vi "Airmar Interpret NMEA Sentence.vi"(11 "NMEA Sentence":string) -> ()   [LabVIEW 2013]
doc: "Interprets the NMEA 0813 sentences that we are using from our Airmar PB200 WeatherStation sensor.\nBy Jaime McCandless\nTODO: finish implementing NMEA sentences"
uses:
  <vilib>/regexp/Match Regular Expression.xnode
  trunk/Software/2-Think/2 Globals/2 Global.vi
  Data/TypeDefs/UTM Location.ctl
  Data/TypeDefs/GPS Sensor Status.ctl
panel:
  out "Estimated error":dbl
  in  "UTC Time Zone":i32=-5
  in  "Tab Control":T1(tab)
  out "GPS (GGA) Data":T2
  out "GPS (GLL) Data":T3
  out "GPGSA Data":T4
  out "UTC Time":timestamp
  out "Local Time":timestamp
  out "Lattitude (ddmm.mmmm)":dbl format="%_8g"
  out "Lattitude North/South":string
  out "Longitude (ddmm.mmmm)":dbl format="%_8g"
  out "Longitude East/West":string
  out "Speed over ground (knots)":dbl format="%_3g"
  out "Course over ground (degrees)":dbl format="%_4g"
  out "Magnetic Variation (degrees)":dbl format="%_4g"
  out "Variation East/West":string
  out "GPS (RMC) Data":T5 {"Course over ground (degrees)" format="%#.6g"; "Speed over ground (knots)" format="%#.6g"; "Magnetic Variation (degrees)" format="%#.6g"; "Longitude (ddmm.mmmm)" format="%#.6g"; "Lattitude (ddmm.mmmm)" format="%#.6g"}
  out "GPS Data Valid?":bool
  out "Robot UTM Location":T6 {"North" format="%#_10f"; "East" format="%#_8f"}
  out "GPS (VTG) Data":T7
  out "Heading":dbl
  out "Turn (ROT) Data":T8
  out "Meteorological Data":T9
  out "Theoretical true wind direction":T10(graph)
  out "Relative wind direction":cluster{dbl, "Filtered Value Out":dbl}(graph)
  out "Wind (MWV) Data, Theoretical":T11
  out "Wind (MWV) Data, Relative":T11
  out "Transducer (XDR) B Data":cluster{"Pitch (deg)":dbl, "Roll (deg)":dbl}
  out "Transducer (XDR) A Data":T12
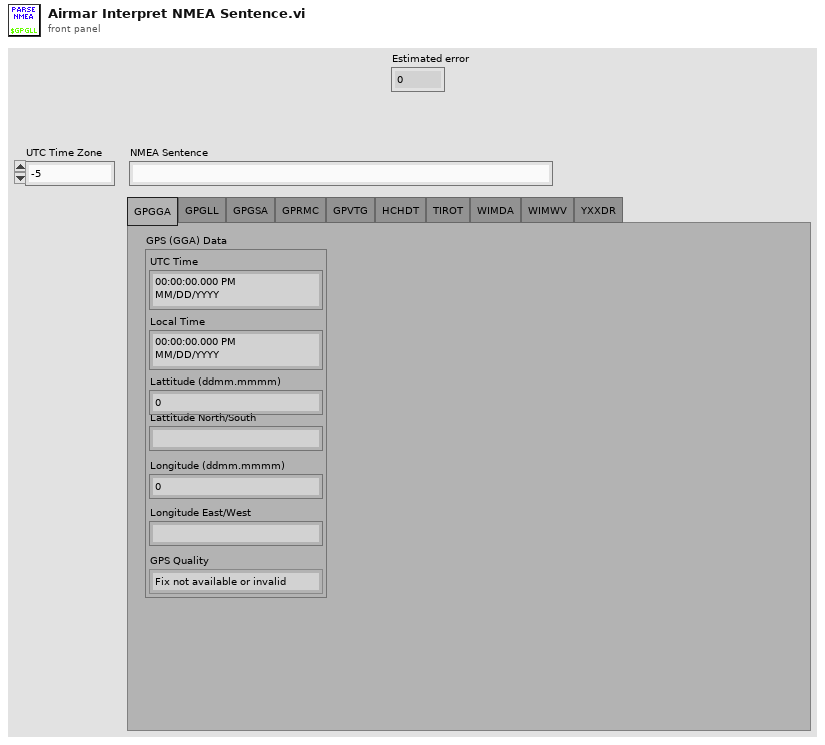
[diagram p1: front panel]
types:
  T1 = enum32{"GPGGA", "GPGLL", "GPGSA", "GPRMC", "GPVTG", "HCHDT", "TIROT", "WIMDA", "WIMWV", "YXXDR"}
  T2 = cluster{"UTC Time":timestamp, "Local Time":timestamp, "Lattitude (ddmm.mmmm)":dbl, "Lattitude North/South":string, "Longitude (ddmm.mmmm)":dbl, "Longitude East/West":string, "GPS Quality":enum16{"Fix not available or invalid", "GPS SPS Mode, fix valid", "Differential GPS, SPS Mode, fix valid", "GPS PPS Mode, fix valid", "Real Time Kinematic (RTK)", "Float RTK", "Estimated (dead reckoning) Mode", "Manual Input Mode", "Simulator Mode"}}
  T3 = cluster{"UTC Time":timestamp, "Local Time":timestamp, "Lattitude (ddmm.mmmm)":dbl, "Lattitude North/South":string, "Longitude (ddmm.mmmm)":dbl, "Longitude East/West":string, "GPS Mode":string, "GPS Data Valid?":bool}
  T4 = cluster{"Mode":string, "Fix Strength":i32, "Satellite IDs":i32[], "PDOP":dbl, "HDOP":dbl, "VDOP":dbl}
  T5 = cluster{"UTC Time":timestamp, "Local Time":timestamp, "Lattitude (ddmm.mmmm)":dbl, "Lattitude North/South":string, "Longitude (ddmm.mmmm)":dbl, "Longitude East/West":string, "Magnetic Variation (degrees)":dbl, "Variation East/West":string, "Speed over ground (knots)":dbl, "Course over ground (degrees)":dbl}
  T6 = typedef "UTM Location.ctl" = cluster{"UTM Zone":dbl, "Hemisphere":enum16{"North", "South"}, "East":dbl, "North":dbl}
  T7 = cluster{"Course Over Ground (True)":dbl, "Course Over Ground (Magnetic)":dbl, "Speed Over Ground (Knots)":dbl, "Speed Over Ground (km/hr)":dbl, "GPS Mode":string}
  T8 = cluster{"Rate of Turn (deg/min)":dbl, "Turn Rotation Data Valid?":bool}
  T9 = cluster{"Barometric Pressure (inches of mercury)":dbl, "Barometric Pressure (bars)":dbl, "Air temperature (degC)":dbl, "Relative humidity (%)":dbl, "Wind direction, True (deg)":dbl, "Wind direction, Magnetic (deg)":dbl, "Wind speed (knots)":dbl, "Wind speed (m/s)":dbl}
  T10 = cluster{"Robot\nHeading ":dbl, "Robot\nHeading ":dbl}
  T11 = cluster{"Angle relative to boat (deg)":dbl, "Wind Data Valid?":bool, "Wind speed (knots)":dbl, "True (T) or Relative (R)":string}
  T12 = cluster{"Calc. Relative Wind Chill (degC)":dbl, "Calc. Theoretical Wind Chill (degC)":dbl, "Calc. Heat Index (degC)":dbl, "Meas. Barometric Pressure (bars)":dbl}
  T13 = cluster{"second":i32, "minute":i32, "hour":i32, "day of month":i32, "month":i32, "year":i32, "day of week":i32, "day of year":i32, "is DST":i32}
  T14 = typedef "GPS Sensor Status.ctl" = cluster{"Sensor Connected":bool, "Sensor OK":bool, "GPS Lock":bool, "Sensor Initialized":bool}
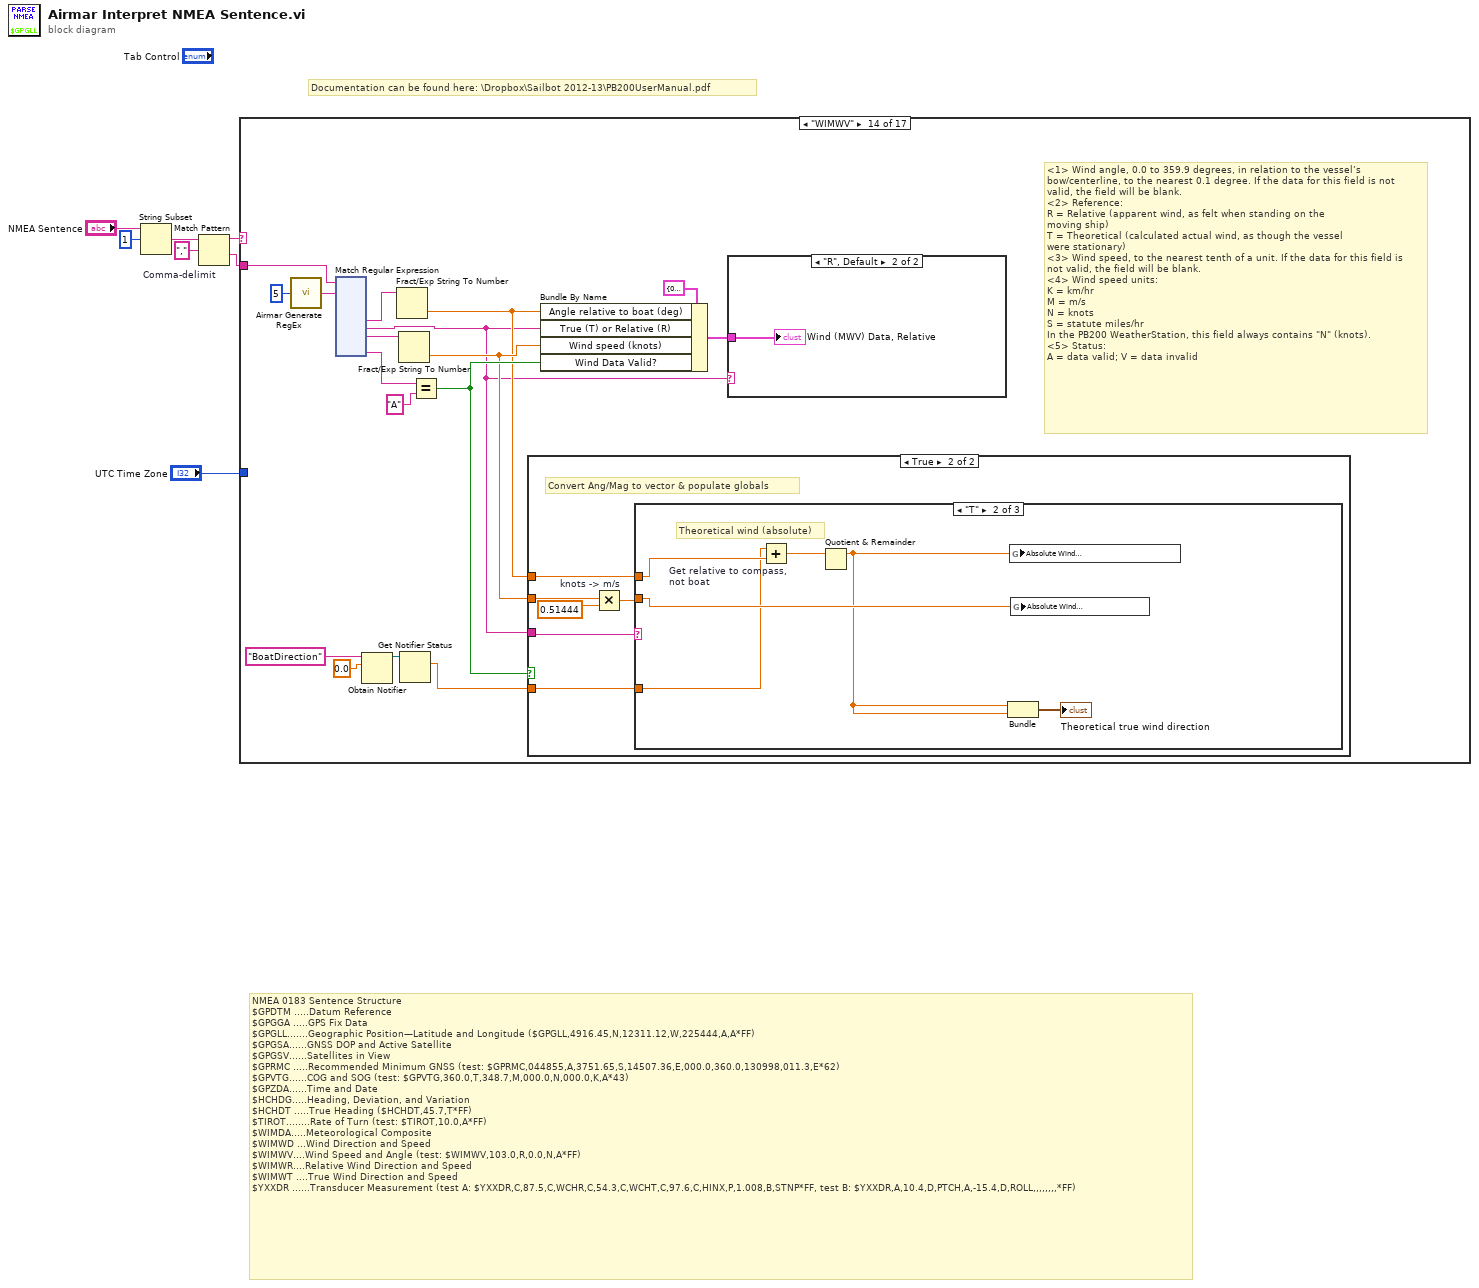
[diagram p0: block diagram]
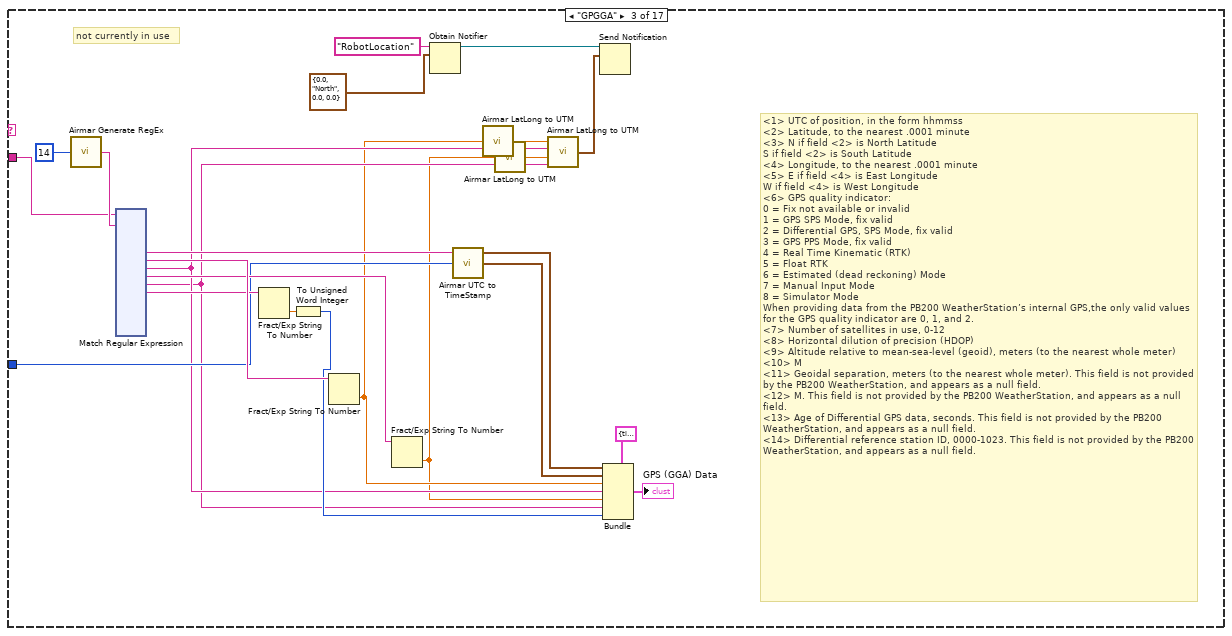
[diagram p4: hidden frame]
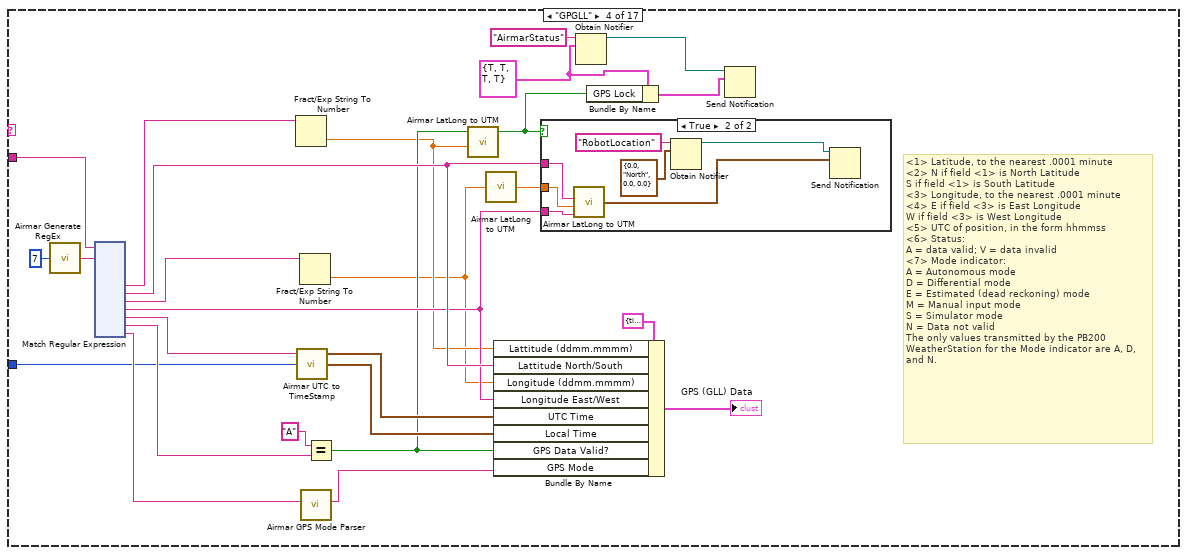
[diagram p5: hidden frame]
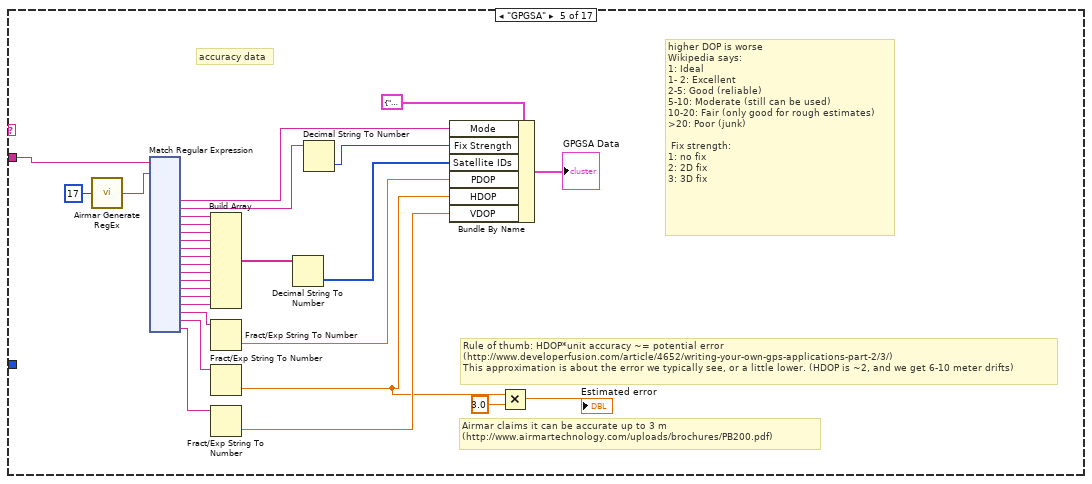
[diagram p7: hidden frame]
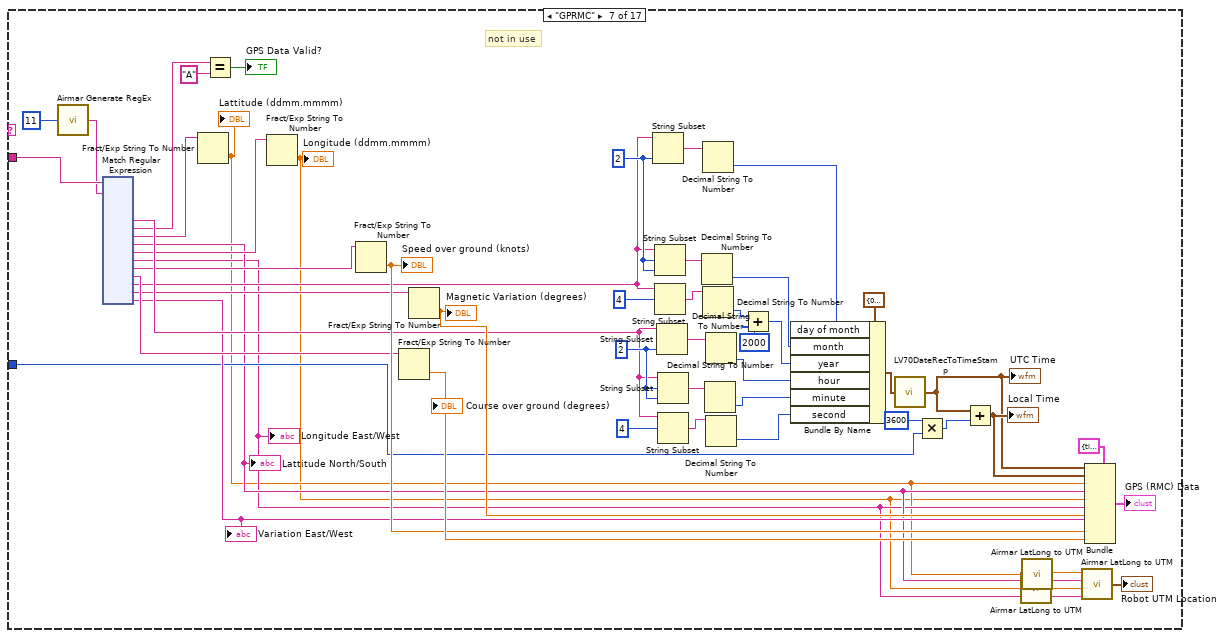
[diagram p9: hidden frame]
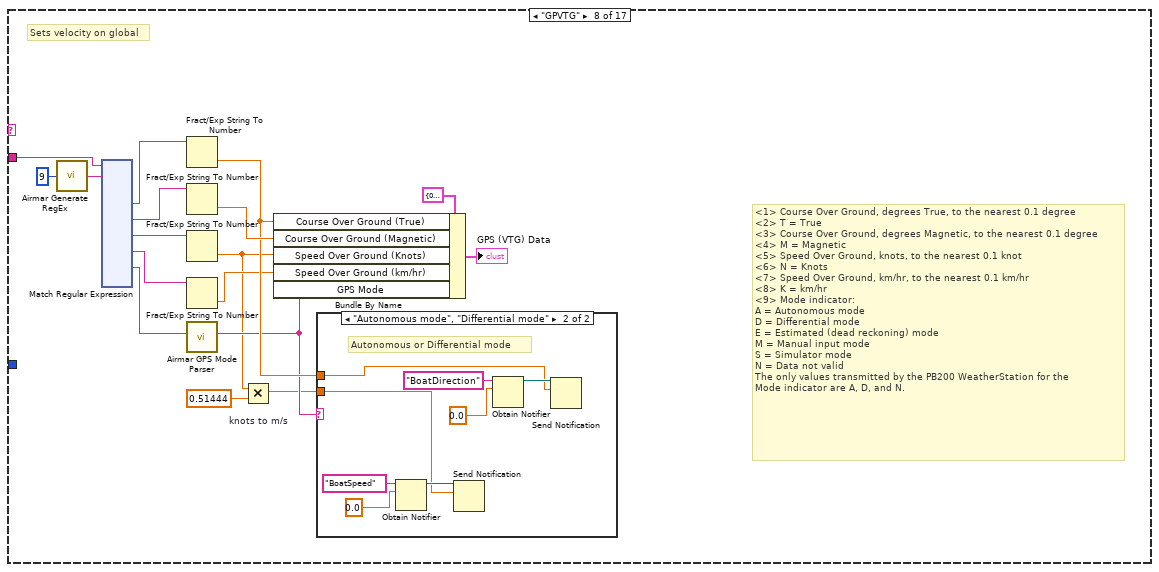
[diagram p10: hidden frame]
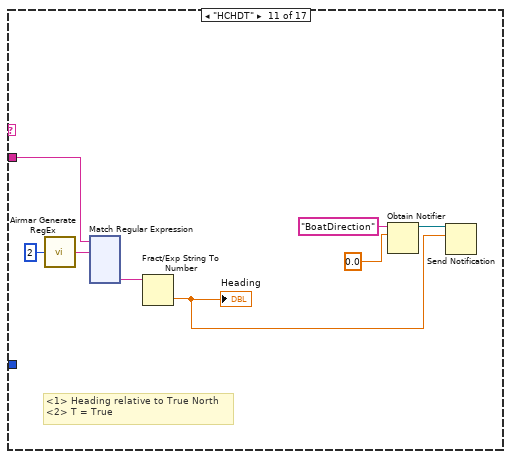
[diagram p14: hidden frame]
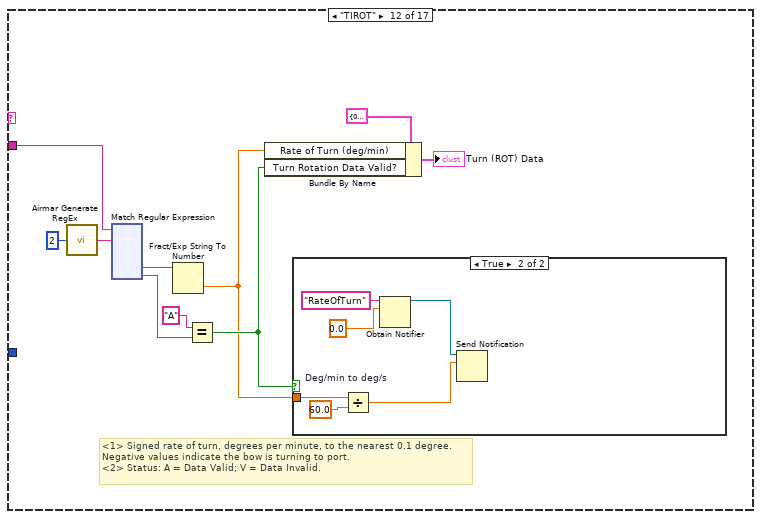
[diagram p15: hidden frame]
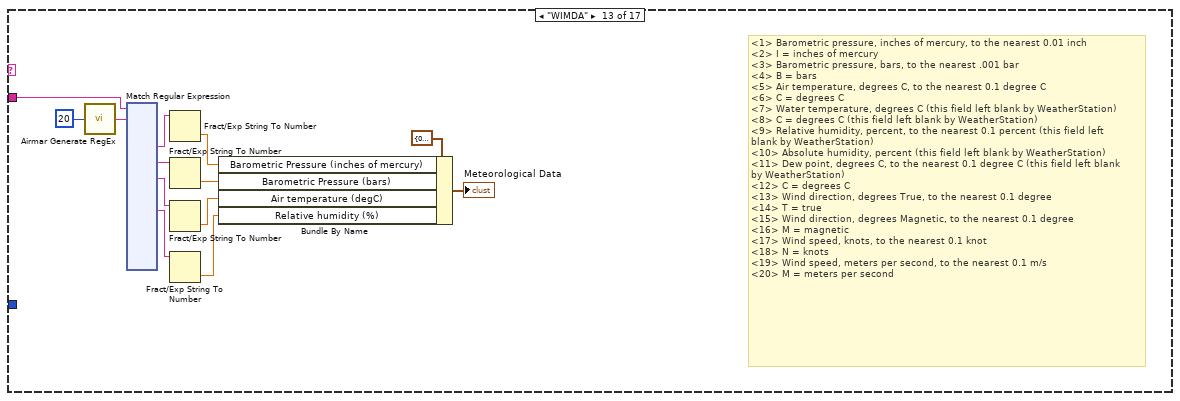
[diagram p17: hidden frame]
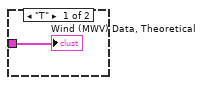
[diagram p18: hidden frame]
diagram:
  # "Documentation can be found here: \\Dropbox\\Sailbot 2012-13\\PB200UserManual.pdf"
  # "NMEA 0183 Sentence Structure\n$GPDTM .....Datum Reference\n$GPGGA .....GPS Fix Data\n$GPGLL.......Geographic Position—Latitude and Longitude ($GPGLL,4916.45,N,12311.12,W,225444,A,A*FF)\n$GPGSA......GNSS DOP and Active Satellite\n$GPGSV......Satellites in View\n$GPRMC .....Recommended Minimum GNSS (test: $GPRMC,044855,A,3751.65,S,14507.36,E,000.0,360.0,130998,011.3,E*62)\n$GPVTG......COG and SOG (test: $GPVTG,360.0,T,348.7,M,000.0,N,000.0,K,A*43)\n$GPZDA......Time and Date\n$HCHDG.....Heading, Deviation, and Variation\n$HCHDT .....True Heading ($HCHDT,45.7,T*FF)\n$TIROT........Rate of Turn (test: $TIROT,10.0,A*FF)\n$WIMDA.....Meteorological Composite\n$WIMWD ...Wind Direction and Speed\n$WIMWV....Wind Speed and Angle (test: $WIMWV,103.0,R,0.0,N,A*FF)\n$WIMWR....Relative Wind Direction and Speed\n$WIMWT ....True Wind Direction and Speed\n$YXXDR ......Transducer Measurement (test A: $YXXDR,C,87.5,C,WCHR,C,54.3,C,WCHT,C,97.6,C,HINX,P,1.008,B,STNP*FF, test B: $YXXDR,A,10.4,D,PTCH,A,-15.4,D,ROLL,,,,,,,,*FF)"
  n1 = String Subset(string="NMEA Sentence", offset (0)=1) -> (substring=w4:string)  [unwired: 1 in]
  n2 = Match Pattern "Comma-delimit"(string=w4, regular expression=",") -> (before substring=w5:string, after substring=w6:string)  [unwired: 1 in, 2 out]
  n3 = case shown="\"WIMWV\"" w5 {
    tunnel: w6 -> [_ _ w29 w174 w335 _ w484 w653 _ _ w792 w914 w1048 w1191 _ _ w1330]
    tunnel: "UTC Time Zone" -> [_ _ w18 w166 _ _ w472 _ _ _ _ _ _ _ _ _ _]
    frame "", Default {
    }
    frame "GPDTM" {
      # "unimplemented"
    }
    frame "GPGGA" {
      # "not currently in use"
      # "<1> UTC of position, in the form hhmmss\n<2> Latitude, to the nearest .0001 minute\n<3> N if field <2> is North Latitude\nS if field <2> is South Latitude\n<4> Longitude, to the nearest .0001 minute\n<5> E if field <4> is East Longitude\nW if field <4> is West Longitude\n<6> GPS quality indicator:\n0 = Fix not available or invalid\n1 = GPS SPS Mode, fix valid\n2 = Differential GPS, SPS Mode, fix valid\n3 = GPS PPS Mode, fix valid\n4 = Real Time Kinematic (RTK)\n5 = Float RTK\n6 = Estimated (dead reckoning) Mode\n7 = Manual Input Mode\n8 = Simulator Mode\nWhen providing data from the PB200 WeatherStation’s internal GPS,the only valid values for the GPS quality indicator are 0, 1, and 2.\n<7> Number of satellites in use, 0-12\n<8> Horizontal dilution of precision (HDOP)\n<9> Altitude relative to mean-sea-level (geoid), meters (to the nearest whole meter)\n<10> M\n<11> Geoidal separation, meters (to the nearest whole meter). This field is not provided by the PB200 WeatherStation, and appears as a null field.\n<12> M. This field is not provided by the PB200 WeatherStation, and appears as a null field.\n<13> Age of Differential GPS data, seconds. This field is not provided by the PB200 WeatherStation, and appears as a null field.\n<14> Differential reference station ID, 0000-1023. This field is not provided by the PB200 WeatherStation, and appears as a null field."
      n4 = call "Airmar Generate RegEx.vi"("# Datums"=14) -> ("RegEx"=w30:string)
      n5 = xnode "Match Regular Expression"("input string"=w29, "regular expression"=w30) -> ("submatch 1"=w21:string, "submatch 2"=w27:string, "submatch 3"=w17:string, "submatch 4"=w26:string, "submatch 5"=w16:string, "submatch 6"=w25:string)  [unwired: 4 in, 10 out]
      n6 = Fract/Exp String To Number(string=w25) -> (number=w24:dbl)  [unwired: 3 in, 1 out]
      n7 = To Unsigned Word Integer(number=w24) -> (unsigned 16bit integer=w23:u16)
      n8 = Fract/Exp String To Number(string=w27) -> (number=w14:dbl)  [unwired: 3 in, 1 out]
      n9 = Fract/Exp String To Number(string=w26) -> (number=w12:dbl)  [unwired: 3 in, 1 out]
      n10 = Obtain Notifier(name (unnamed)="RobotLocation", notification data type=T6 {"UTM Zone"=0.0, "Hemisphere"=enum."North", "East"=0.0, "North"=0.0} ("UTM Location")) -> (notifier out=w9:refnum<notifier>)  [unwired: 2 in, 2 out]
      n11 = call "Airmar UTC to TimeStamp.vi"("UTC Time Zone in"=w18, "UTC (hhmmss)"=w21) -> ("Local Time"=w19:timestamp, "UTC Time"=w20:timestamp)  [unwired: 2 in]
      n12 = call "Airmar LatLong to UTM.vi"("Lattitude/Longitude in ddmm.mmmm"=w14) -> ("Latitude/Longitude in dd.dddddd"=w15:dbl)
      n13 = call "Airmar LatLong to UTM.vi"("Lattitude/Longitude in ddmm.mmmm"=w12) -> ("Latitude/Longitude in dd.dddddd"=w13:dbl)
      n14 = call "Airmar LatLong to UTM.vi"("East/West"=w16, "Longitude"=w13, "North/South"=w17, "Latitude"=w15) -> ("Robot UTM Location"=w8:T6)
      n15 = Send Notification(notification=w8, notifier=w9) -> ()  [unwired: 1 in, 2 out]
      n16 = Bundle(cluster=T2 {"UTC Time"=timestamp(0 s since 1904-01-01), "Local Time"=timestamp(0 s since 1904-01-01), "Lattitude (ddmm.mmmm)"=0.0, "Lattitude North/South"="", "Longitude (ddmm.mmmm)"=0.0, "Longitude East/West"="", "GPS Quality"=enum."GPS SPS Mode, fix valid"} ("Cluster"), "UTC Time"=w20, "Local Time"=w19, "Lattitude (ddmm.mmmm)"=w14, "Lattitude North/South"=w17, "Longitude (ddmm.mmmm)"=w12, "Longitude East/West"=w16, "GPS Quality"=w23) -> (→"GPS (GGA) Data":T2)
    }
    frame "GPGLL" {
      w157 = T14 {"Sensor Connected"=TRUE, "Sensor OK"=TRUE, "GPS Lock"=TRUE, "Sensor Initialized"=TRUE} ("input cluster")
      # "<1> Latitude, to the nearest .0001 minute\n<2> N if field <1> is North Latitude\nS if field <1> is South Latitude\n<3> Longitude, to the nearest .0001 minute\n<4> E if field <3> is East Longitude\nW if field <3> is West Longitude\n<5> UTC of position, in the form hhmmss\n<6> Status:\nA = data valid; V = data invalid\n<7> Mode indicator:\nA = Autonomous mode\nD = Differential mode\nE = Estimated (dead reckoning) mode\nM = Manual input mode\nS = Simulator mode\nN = Data not valid\nThe only values transmitted by the PB200 WeatherStation for the Mode indicator are A, D, and N."
      n17 = call "Airmar Generate RegEx.vi"("# Datums"=7) -> ("RegEx"=w178:string)
      n18 = xnode "Match Regular Expression"("input string"=w174, "regular expression"=w178) -> ("submatch 1"=w177:string, "submatch 2"=w164:string, "submatch 3"=w176:string, "submatch 4"=w163:string, "submatch 5"=w173:string, "submatch 6"=w169:string, "submatch 7"=w175:string)  [unwired: 4 in, 5 out]
      n19 = Fract/Exp String To Number(string=w177) -> (number=w161:dbl)  [unwired: 3 in, 1 out]
      n20 = call "Airmar UTC to TimeStamp.vi"("UTC Time Zone in"=w166, "UTC (hhmmss)"=w173) -> ("Local Time"=w168:timestamp, "UTC Time"=w167:timestamp)  [unwired: 2 in]
      n21 = Fract/Exp String To Number(string=w176) -> (number=w160:dbl)  [unwired: 3 in, 1 out]
      n22 = call "Airmar GPS Mode Parser.vi"("GPS Mode (Char)"=w175) -> ("GPS Mode (Description)"=w171:string)  [unwired: 6 in]
      n23 = Equal?(x="A" ("y"), y=w169) -> (x = y?=w162:bool)
      n24 = call "Airmar LatLong to UTM.vi"("Longitude"=w161) -> ()  [unwired: 3 in, 1 out]
      n25 = call "Airmar LatLong to UTM.vi"("Lattitude/Longitude in ddmm.mmmm"=w160) -> ("Latitude/Longitude in dd.dddddd"=w159:dbl)
      n26 = Bundle By Name(cluster=T3 {"UTC Time"=timestamp(0 s since 1904-01-01), "Local Time"=timestamp(0 s since 1904-01-01), "Lattitude (ddmm.mmmm)"=0.0, "Lattitude North/South"="", "Longitude (ddmm.mmmm)"=0.0, "Longitude East/West"="", "GPS Mode"="", "GPS Data Valid?"=FALSE} ("Cluster"), "Lattitude (ddmm.mmmm)"=w161, "Lattitude North/South"=w164, "Longitude (ddmm.mmmm)"=w160, "Longitude East/West"=w163, "UTC Time"=w167, "Local Time"=w168, "GPS Data Valid?"=w162, "GPS Mode"=w171) -> (→"GPS (GLL) Data":T3)
      n27 = case shown="True" w162 {
        tunnel: w164 -> [_ w186]
        tunnel: w159 -> [_ w185]
        tunnel: w163 -> [_ w184]
        frame False {
        }
        frame True {
          n28 = call "Airmar LatLong to UTM.vi"("East/West"=w184, "Longitude"=w185, "North/South"=w186) -> ("Robot UTM Location"=w183:T6)  [unwired: 1 in]
          n29 = Obtain Notifier(name (unnamed)="RobotLocation", notification data type=T6 {"UTM Zone"=0.0, "Hemisphere"=enum."North", "East"=0.0, "North"=0.0} ("UTM Location")) -> (notifier out=w180:refnum<notifier>)  [unwired: 2 in, 2 out]
          n30 = Send Notification(notification=w183, notifier=w180) -> ()  [unwired: 1 in, 2 out]
        }
      }
      n31 = Obtain Notifier(name (unnamed)="AirmarStatus", notification data type=w157) -> (notifier out=w156:refnum<notifier>)  [unwired: 2 in, 2 out]
      n32 = Bundle By Name(cluster=w157, "GPS Lock"=w162) -> (w155:T14)
      n33 = Send Notification(notification=w155, notifier=w156) -> ()  [unwired: 1 in, 2 out]
    }
    frame "GPGSA" {
      # "Airmar claims it can be accurate up to 3 m\n(http://www.airmartechnology.com/uploads/brochures/PB200.pdf)"
      # "Rule of thumb: HDOP*unit accuracy ~= potential error\n(http://www.developerfusion.com/article/4652/writing-your-own-gps-applications-part-2/3/)\nThis approximation is about the error we typically see, or a little lower. (HDOP is ~2, and we get 6-10 meter drifts)"
      # "higher DOP is worse\nWikipedia says:\n1: Ideal\n1- 2: Excellent\n2-5: Good (reliable)\n5-10: Moderate (still can be used)\n10-20: Fair (only good for rough estimates)\n>20: Poor (junk)\n\n Fix strength: \n1: no fix\n2: 2D fix\n3: 3D fix"
      # "accuracy data"
      n34 = call "Airmar Generate RegEx.vi"("# Datums"=17) -> ("RegEx"=w334:string)
      n35 = xnode "Match Regular Expression"("input string"=w335, "regular expression"=w334) -> ("submatch 1"=w331:string, "submatch 2"=w330:string, "submatch 3"=w328:string, "submatch 4"=w327:string, "submatch 5"=w326:string, "submatch 6"=w325:string, "submatch 7"=w324:string, "submatch 8"=w323:string, "submatch 9"=w322:string, "submatch 10"=w321:string, "submatch 11"=w320:string, "submatch 12"=w319:string, "submatch 13"=w318:string, "submatch 14"=w317:string, "submatch 15"=w314:string, "submatch 16"=w312:string, "submatch 17"=w311:string)  [unwired: 4 in, 5 out]
      n36 = Build Array(w328, w327, w326, w325, w324, w323, w322, w321, w320, w319, w318, w317) -> (w316:string[])
      n37 = Fract/Exp String To Number(string=w314) -> (number=w313:dbl)  [unwired: 3 in, 1 out]
      n38 = Fract/Exp String To Number(string=w312) -> (number=w308:dbl)  [unwired: 3 in, 1 out]
      n39 = Fract/Exp String To Number(string=w311) -> (number=w310:dbl)  [unwired: 3 in, 1 out]
      n40 = Decimal String To Number(string=w316) -> (number=w315:i32[])  [unwired: 2 in, 1 out]
      n41 = Decimal String To Number(string=w330) -> (number=w329:i32)  [unwired: 2 in, 1 out]
      n42 = Bundle By Name(cluster=T4 {"Mode"="", "Fix Strength"=0, "Satellite IDs"=[], "PDOP"=0.0, "HDOP"=0.0, "VDOP"=0.0} ("GPGSA Data"), "Mode"=w331, "Fix Strength"=w329, "Satellite IDs"=w315, "PDOP"=w313, "HDOP"=w308, "VDOP"=w310) -> (→"GPGSA Data":T4)
      n43 = Multiply(x=w308, y=3.0) -> (x*y=→"Estimated error":dbl)
    }
    frame "GPGSV" {
      # "unimplemented"
    }
    frame "GPRMC" {
      w502 = 2 ("length (rest)")
      w492 = 2 ("length (rest)")
      # "not in use"
      n44 = call "Airmar Generate RegEx.vi"("# Datums"=11) -> ("RegEx"=w474:string)
      n45 = xnode "Match Regular Expression"("input string"=w484, "regular expression"=w474) -> ("submatch 1"=w483:string, "submatch 2"=w482:string, "submatch 3"=w481:string, "submatch 4"=w471:string, "submatch 5"=w480:string, "submatch 6"=w470:string, "submatch 7"=w479:string, "submatch 8"=w478:string, "submatch 9"=w477:string, "submatch 10"=w476:string, "submatch 11"=w475:string)  [unwired: 4 in, 5 out]
      "Lattitude North/South" <- w471
      "Longitude East/West" <- w470
      "Variation East/West" <- w475
      n46 = Fract/Exp String To Number(string=w481) -> (number=w467:dbl)  [unwired: 3 in, 1 out]
      "Lattitude (ddmm.mmmm)" <- w467
      n47 = Equal?(x=w482, y="A") -> (x = y?=→"GPS Data Valid?":bool)
      n48 = Fract/Exp String To Number(string=w480) -> (number=w465:dbl)  [unwired: 3 in, 1 out]
      "Longitude (ddmm.mmmm)" <- w465
      n49 = Fract/Exp String To Number(string=w479) -> (number=w512:dbl)  [unwired: 3 in, 1 out]
      "Speed over ground (knots)" <- w512
      n50 = Fract/Exp String To Number(string=w478) -> (number=w513:dbl)  [unwired: 3 in, 1 out]
      "Course over ground (degrees)" <- w513
      n51 = Fract/Exp String To Number(string=w476) -> (number=w511:dbl)  [unwired: 3 in, 1 out]
      "Magnetic Variation (degrees)" <- w511
      n52 = String Subset(string=w477, length (rest)=w502) -> (substring=w503:string)  [unwired: 1 in]
      n53 = String Subset(string=w477, offset (0)=w502, length (rest)=w502) -> (substring=w501:string)
      n54 = String Subset(string=w477, offset (0)=4) -> (substring=w499:string)  [unwired: 1 in]
      n55 = String Subset(string=w483, length (rest)=w492) -> (substring=w488:string)  [unwired: 1 in]
      n56 = String Subset(string=w483, offset (0)=w492, length (rest)=w492) -> (substring=w494:string)
      n57 = String Subset(string=w483, offset (0)=4) -> (substring=w496:string)  [unwired: 1 in]
      n58 = Decimal String To Number(string=w501) -> (number=w505:i32)  [unwired: 2 in, 1 out]
      n59 = Decimal String To Number(string=w503) -> (number=w504:i32)  [unwired: 2 in, 1 out]
      n60 = Decimal String To Number(string=w499) -> (number=w506:i32)  [unwired: 2 in, 1 out]
      n61 = Decimal String To Number(string=w494) -> (number=w493:i32)  [unwired: 2 in, 1 out]
      n62 = Decimal String To Number(string=w488) -> (number=w491:i32)  [unwired: 2 in, 1 out]
      n63 = Decimal String To Number(string=w496) -> (number=w497:i32)  [unwired: 2 in, 1 out]
      n64 = Add(x=w506, y=2000) -> (x+y=w508:i32)
      n65 = Bundle By Name(cluster=T13 {"second"=0, "minute"=0, "hour"=0, "day of month"=0, "month"=0, "year"=0, "day of week"=0, "day of year"=0, "is DST"=0} ("date time rec"), "day of month"=w504, "month"=w505, "year"=w508, "hour"=w491, "minute"=w493, "second"=w497) -> (w489:T13)
      n66 = call <vilib>:"LV70DateRecToTimeStamp.vi"("date time rec"=w489) -> ("Time Stamp"=w509:timestamp)
      "UTC Time" <- w509
      n67 = Multiply(x=3600 ("number"), y=w472) -> (x*y=w473:i32)
      n68 = Add(x=w509, y=w473) -> (x+y=w510:timestamp)
      "Local Time" <- w510
      n69 = call "Airmar LatLong to UTM.vi"("Lattitude/Longitude in ddmm.mmmm"=w465) -> ("Latitude/Longitude in dd.dddddd"=w466:dbl)
      n70 = call "Airmar LatLong to UTM.vi"("Lattitude/Longitude in ddmm.mmmm"=w467) -> ("Latitude/Longitude in dd.dddddd"=w468:dbl)
      n71 = call "Airmar LatLong to UTM.vi"("East/West"=w470, "Longitude"=w466, "North/South"=w471, "Latitude"=w468) -> ("Robot UTM Location"=→"Robot UTM Location":T6)
      n72 = Bundle(cluster=T5 {"UTC Time"=timestamp(0 s since 1904-01-01), "Local Time"=timestamp(0 s since 1904-01-01), "Lattitude (ddmm.mmmm)"=0.0, "Lattitude North/South"="", "Longitude (ddmm.mmmm)"=0.0, "Longitude East/West"="", "Magnetic Variation (degrees)"=0.0, "Variation East/West"="", "Speed over ground (knots)"=0.0, "Course over ground (degrees)"=0.0} ("Cluster"), "UTC Time"=w509, "Local Time"=w510, "Lattitude (ddmm.mmmm)"=w467, "Lattitude North/South"=w471, "Longitude (ddmm.mmmm)"=w465, "Longitude East/West"=w470, "Magnetic Variation (degrees)"=w511, "Variation East/West"=w475, "Speed over ground (knots)"=w512, "Course over ground (degrees)"=w513) -> (→"GPS (RMC) Data":T5)
    }
    frame "GPVTG" {
      # "Sets velocity on global"
      # "<1> Course Over Ground, degrees True, to the nearest 0.1 degree\n<2> T = True\n<3> Course Over Ground, degrees Magnetic, to the nearest 0.1 degree\n<4> M = Magnetic\n<5> Speed Over Ground, knots, to the nearest 0.1 knot\n<6> N = Knots\n<7> Speed Over Ground, km/hr, to the nearest 0.1 km/hr\n<8> K = km/hr\n<9> Mode indicator:\nA = Autonomous mode\nD = Differential mode\nE = Estimated (dead reckoning) mode\nM = Manual input mode\nS = Simulator mode\nN = Data not valid\nThe only values transmitted by the PB200 WeatherStation for the\nMode indicator are A, D, and N."
      n73 = call "Airmar Generate RegEx.vi"("# Datums"=9) -> ("RegEx"=w654:string)
      n74 = xnode "Match Regular Expression"("input string"=w653, "regular expression"=w654) -> ("submatch 1"=w650:string, "submatch 3"=w649:string, "submatch 5"=w647:string, "submatch 7"=w646:string, "submatch 9"=w645:string)  [unwired: 4 in, 11 out]
      n75 = Fract/Exp String To Number(string=w650) -> (number=w644:dbl)  [unwired: 3 in, 1 out]
      n76 = Fract/Exp String To Number(string=w649) -> (number=w648:dbl)  [unwired: 3 in, 1 out]
      n77 = Fract/Exp String To Number(string=w647) -> (number=w641:dbl)  [unwired: 3 in, 1 out]
      n78 = Fract/Exp String To Number(string=w646) -> (number=w643:dbl)  [unwired: 3 in, 1 out]
      n79 = call "Airmar GPS Mode Parser.vi"("GPS Mode (Char)"=w645) -> ("GPS Mode (Description)"=w642:string)  [unwired: 6 in]
      n80 = Multiply "knots to m/s"(x=w641, y=0.51444) -> (x*y=w640:dbl)
      n81 = Bundle By Name(cluster=T7 {"Course Over Ground (True)"=0.0, "Course Over Ground (Magnetic)"=0.0, "Speed Over Ground (Knots)"=0.0, "Speed Over Ground (km/hr)"=0.0, "GPS Mode"=""} ("GPS (VTG) Data 2"), "Course Over Ground (True)"=w644, "Course Over Ground (Magnetic)"=w648, "Speed Over Ground (Knots)"=w641, "Speed Over Ground (km/hr)"=w643, "GPS Mode"=w642) -> (→"GPS (VTG) Data":T7)
      n82 = case shown="\"Autonomous mode\", \"Differential mode\"" w642 {
        tunnel: w644 -> [_ w657]
        tunnel: w640 -> [_ w661]
        frame "Data not valid", Default {
          # "Data not valid"
        }
        frame "Autonomous mode", "Differential mode" {
          # "Autonomous or Differential mode"
          n83 = Obtain Notifier(name (unnamed)="BoatSpeed", notification data type=0.0 ("number")) -> (notifier out=w663:refnum<notifier>)  [unwired: 2 in, 2 out]
          n84 = Send Notification(notification=w661, notifier=w663) -> ()  [unwired: 1 in, 2 out]
          n85 = Obtain Notifier(name (unnamed)="BoatDirection", notification data type=0.0 ("number")) -> (notifier out=w659:refnum<notifier>)  [unwired: 2 in, 2 out]
          n86 = Send Notification(notification=w657, notifier=w659) -> ()  [unwired: 1 in, 2 out]
        }
      }
    }
    frame "GPZDA" {
      # "<1> UTC time of day, in the form hhmmss\n<2> UTC day, 01 to 31\n<3> UTC month, 01 to 12\n<4> UTC year (four digits, e.g. 2006)\n<5> Local time zone hours, 00 to +/-13 hrs\n<6> Local time zone minutes, 00 to +59"
    }
    frame "HCHDG " {
      # "<1> Magnetic sensor heading, degrees, to the nearest 0.1 degree.\n<2> Magnetic deviation, degrees east or west, to the nearest 0.1 degree.\n<3> E if field <2> is degrees East\nW if field <2> is degrees West\n<4> Magnetic variation, degrees east or west, to the nearest 0.1 degree.\n<5> E if field <4> is degrees East\nW if field <4> is degrees West"
    }
    frame "HCHDT" {
      # "<1> Heading relative to True North\n<2> T = True"
      n87 = call "Airmar Generate RegEx.vi"("# Datums"=2) -> ("RegEx"=w793:string)
      n88 = xnode "Match Regular Expression"("input string"=w792, "regular expression"=w793) -> ("submatch 1"=w791:string)  [unwired: 4 in, 5 out]
      n89 = Fract/Exp String To Number(string=w791) -> (number=w787:dbl)  [unwired: 3 in, 1 out]
      "Heading" <- w787
      n90 = Obtain Notifier(name (unnamed)="BoatDirection", notification data type=0.0 ("number")) -> (notifier out=w790:refnum<notifier>)  [unwired: 2 in, 2 out]
      n91 = Send Notification(notification=w787, notifier=w790) -> ()  [unwired: 1 in, 2 out]
    }
    frame "TIROT" {
      # "<1> Signed rate of turn, degrees per minute, to the nearest 0.1 degree.\nNegative values indicate the bow is turning to port.\n<2> Status: A = Data Valid; V = Data Invalid."
      n92 = call "Airmar Generate RegEx.vi"("# Datums"=2) -> ("RegEx"=w916:string)
      n93 = xnode "Match Regular Expression"("input string"=w914, "regular expression"=w916) -> ("submatch 1"=w915:string, "submatch 2"=w910:string)  [unwired: 4 in, 5 out]
      n94 = Fract/Exp String To Number(string=w915) -> (number=w908:dbl)  [unwired: 3 in, 1 out]
      n95 = Equal?(x="A" ("y"), y=w910) -> (x = y?=w909:bool)
      n96 = Bundle By Name(cluster=T8 {"Rate of Turn (deg/min)"=0.0, "Turn Rotation Data Valid?"=TRUE} ("Turn (ROT) Data 2"), "Rate of Turn (deg/min)"=w908, "Turn Rotation Data Valid?"=w909) -> (→"Turn (ROT) Data":T8)
      n97 = case shown="True" w909 {
        tunnel: w908 -> [_ w923]
        frame False {
        }
        frame True {
          n98 = Divide "Deg/min to deg/s"(x=w923, y=60.0) -> (x/y=w919:dbl)
          n99 = Obtain Notifier(name (unnamed)="RateOfTurn", notification data type=0.0) -> (notifier out=w918:refnum<notifier>)  [unwired: 2 in, 2 out]
          n100 = Send Notification(notification=w919, notifier=w918) -> ()  [unwired: 1 in, 2 out]
        }
      }
    }
    frame "WIMDA" {
      # "<1> Barometric pressure, inches of mercury, to the nearest 0.01 inch\n<2> I = inches of mercury\n<3> Barometric pressure, bars, to the nearest .001 bar\n<4> B = bars\n<5> Air temperature, degrees C, to the nearest 0.1 degree C\n<6> C = degrees C\n<7> Water temperature, degrees C (this field left blank by WeatherStation)\n<8> C = degrees C (this field left blank by WeatherStation)\n<9> Relative humidity, percent, to the nearest 0.1 percent (this field left\nblank by WeatherStation)\n<10> Absolute humidity, percent (this field left blank by WeatherStation)\n<11> Dew point, degrees C, to the nearest 0.1 degree C (this field left blank\nby WeatherStation)\n<12> C = degrees C\n<13> Wind direction, degrees True, to the nearest 0.1 degree\n<14> T = true\n<15> Wind direction, degrees Magnetic, to the nearest 0.1 degree\n<16> M = magnetic\n<17> Wind speed, knots, to the nearest 0.1 knot\n<18> N = knots\n<19> Wind speed, meters per second, to the nearest 0.1 m/s\n<20> M = meters per second"
      n101 = call "Airmar Generate RegEx.vi"("# Datums"=20) -> ("RegEx"=w1049:string)
      n102 = xnode "Match Regular Expression"("input string"=w1048, "regular expression"=w1049) -> ("submatch 1"=w1042:string, "submatch 3"=w1041:string, "submatch 5"=w1040:string, "submatch 9"=w1039:string)  [unwired: 4 in, 17 out]
      n103 = Fract/Exp String To Number(string=w1042) -> (number=w1046:dbl)  [unwired: 3 in, 1 out]
      n104 = Fract/Exp String To Number(string=w1041) -> (number=w1045:dbl)  [unwired: 3 in, 1 out]
      n105 = Fract/Exp String To Number(string=w1040) -> (number=w1044:dbl)  [unwired: 3 in, 1 out]
      n106 = Fract/Exp String To Number(string=w1039) -> (number=w1043:dbl)  [unwired: 3 in, 1 out]
      n107 = Bundle By Name(cluster=T9 {"Barometric Pressure (inches of mercury)"=0.0, "Barometric Pressure (bars)"=0.0, "Air temperature (degC)"=0.0, "Relative humidity (%)"=0.0, "Wind direction, True (deg)"=0.0, "Wind direction, Magnetic (deg)"=0.0, "Wind speed (knots)"=0.0, "Wind speed (m/s)"=0.0} ("Meteorological Data"), "Barometric Pressure (inches of mercury)"=w1046, "Barometric Pressure (bars)"=w1045, "Air temperature (degC)"=w1044, "Relative humidity (%)"=w1043) -> (→"Meteorological Data":T9)
    }
    frame "WIMWV" {
      # "<1> Wind angle, 0.0 to 359.9 degrees, in relation to the vessel’s\nbow/centerline, to the nearest 0.1 degree. If the data for this field is not\nvalid, the field will be blank.\n<2> Reference:\nR = Relative (apparent wind, as felt when standing on the\nmoving ship)\nT = Theoretical (calculated actual wind, as though the vessel\nwere stationary)\n<3> Wind speed, to the nearest tenth of a unit. If the data for this field is\nnot valid, the field will be blank.\n<4> Wind speed units:\nK = km/hr\nM = m/s\nN = knots\nS = statute miles/hr\nIn the PB200 WeatherStation, this field always contains \"N\" (knots).\n<5> Status:\nA = data valid; V = data invalid"
      n108 = call "Airmar Generate RegEx.vi"("# Datums"=5) -> ("RegEx"=w1194:string)
      n109 = xnode "Match Regular Expression"("input string"=w1191, "regular expression"=w1194) -> ("submatch 1"=w1193:string, "submatch 2"=w1183:string, "submatch 3"=w1188:string, "submatch 5"=w1187:string)  [unwired: 4 in, 6 out]
      n110 = Obtain Notifier(name (unnamed)="BoatDirection", notification data type=0.0) -> (notifier out=w1179:refnum<notifier>)  [unwired: 2 in, 2 out]
      n111 = Fract/Exp String To Number(string=w1193) -> (number=w1184:dbl)  [unwired: 3 in, 1 out]
      n112 = Fract/Exp String To Number(string=w1188) -> (number=w1185:dbl)  [unwired: 3 in, 1 out]
      n113 = Get Notifier Status(notifier=w1179) -> (current notification=w1182:dbl)  [unwired: 1 in, 4 out]
      n114 = Equal?(x=w1187, y="A") -> (x = y?=w1186:bool)
      n115 = case shown="True" w1186 {
        tunnel: w1185 -> [_ w1200]
        tunnel: w1184 -> [_ w1203]
        tunnel: w1183 -> [_ w1202]
        tunnel: w1182 -> [_ w1198]
        frame False {
        }
        frame True {
          # "Convert Ang/Mag to vector & populate globals"
          n116 = Multiply "knots -> m/s"(x=w1200, y=0.51444) -> (x*y=w1201:dbl)
          n117 = case shown="\"T\"" w1202 {
            tunnel: w1201 -> [_ w1207 w1210]
            tunnel: w1203 -> [_ w1209 w1211]
            tunnel: w1198 -> [_ w1204 _]
            frame "", Default {
            }
            frame "T" {
              # "Theoretical wind (absolute)"
              n118 = Add "Get relative to compass, not boat"(x=w1204, y=w1209) -> (x+y=w1208:dbl)
              n119 = Quotient & Remainder(x=w1208) -> (x-y*floor(x/y)=w1206:dbl)  [unwired: 1 in, 1 out]
              n120 = Bundle(w1206, w1206) -> (→"Theoretical true wind direction":cluster{dbl, dbl})  [unwired: 1 in]
              n121 = global write "2 Global.vi" "Absolute Wind\nDirection (º)"(w1206) -> ()
              n122 = global write "2 Global.vi" "Absolute Wind\nSpeed"(w1207) -> ()
            }
            frame "R" {
              # "Relative wind (apparent)"
              n123 = Bundle(w1211, w1211) -> (→"Relative wind direction":cluster{dbl, dbl})  [unwired: 1 in]
              n124 = global write "2 Global.vi" "Apparent Wind\nDirection (º)"(w1211) -> ()
              n125 = global write "2 Global.vi" "Apparent Wind\nSpeed"(w1210) -> ()
            }
          }
        }
      }
      n126 = Bundle By Name(cluster=T11 {"Angle relative to boat (deg)"=0.0, "Wind Data Valid?"=TRUE, "Wind speed (knots)"=0.0, "True (T) or Relative (R)"=""} ("Wind (MWV) Data 2"), "Angle relative to boat (deg)"=w1184, "True (T) or Relative (R)"=w1183, "Wind speed (knots)"=w1185, "Wind Data Valid?"=w1186) -> (w1190:T11)
      n127 = case shown="\"R\", Default" w1183 {
        tunnel: w1190 -> [w1196 w1197]
        frame "T" {
          "Wind (MWV) Data, Theoretical" <- w1196
        }
        frame "R", Default {
          "Wind (MWV) Data, Relative" <- w1197
        }
      }
    }
    frame "WIMWR" {
    }
    frame "WIMWT" {
    }
    frame "YXXDR" {
      n128 = Unbundle By Name() -> ()  [unwired: 1 in, 1 out]
      n129 = String Subset(string=w1330, length (rest)=1 ("length (rest)")) -> (substring=w1331:string)  [unwired: 1 in]
      n130 = case shown="\"A\"" w1331 {
        tunnel: w1330 -> [_ w1341 w1476]
        frame "", Default {
        }
        frame "A" {
          # "TYPE B:\n<1> A = angular displacement\n<2> Pitch: oscillation of vessel about its latitudinal axis. Bow moving up is positive. Value reported to the nearest 0.1 degree.\n<3> D = degrees\n<4> PTCH (ID indicating pitch of vessel)\n<5> A = angular displacement\n<6> Roll: oscillation of vessel about its longitudinal axis. Roll to the starboard is positive. Value reported to the nearest 0.1 degree.\n<7> D = degrees\n<8> ROLL (ID indicating roll of vessel)\n<9> Not used\n<10> Not used\n<11> Not used\n<12> Not used\n<13> Not used\n<14> Not used\n<15> Not used\n<16> Not used"
          n131 = call "Airmar Generate RegEx.vi"("# Datums"=8) -> ("RegEx"=w1345:string)
          n132 = xnode "Match Regular Expression"("input string"=w1341, "regular expression"=w1345) -> ("submatch 2"=w1343:string, "submatch 6"=w1342:string)  [unwired: 4 in, 19 out]
          n133 = Fract/Exp String To Number(string=w1343) -> (number=w1337:dbl)  [unwired: 3 in, 1 out]
          n134 = Fract/Exp String To Number(string=w1342) -> (number=w1334:dbl)  [unwired: 3 in, 1 out]
          n135 = Obtain Notifier(name (unnamed)="Roll", notification data type=0.0 ("number")) -> (notifier out=w1335:refnum<notifier>)  [unwired: 2 in, 2 out]
          n136 = Obtain Notifier(name (unnamed)="Pitch", notification data type=0.0 ("number")) -> (notifier out=w1338:refnum<notifier>)  [unwired: 2 in, 2 out]
          n137 = Bundle By Name(cluster=cluster{"Pitch (deg)":dbl, "Roll (deg)":dbl} {"Pitch (deg)"=103.0, "Roll (deg)"=103.0} ("Transducer (XDR) B Data 2"), "Pitch (deg)"=w1337, "Roll (deg)"=w1334) -> (→"Transducer (XDR) B Data":cluster{"Pitch (deg)":dbl, "Roll (deg)":dbl})
          n138 = Send Notification(notification=w1334, notifier=w1335) -> ()  [unwired: 1 in, 2 out]
          n139 = Send Notification(notification=w1337, notifier=w1338) -> ()  [unwired: 1 in, 2 out]
        }
        frame "C" {
          # "TYPE A:\n<1> C = temperature\n<2> Calculated “relative” wind chill temperature, degrees Celsius, to the nearest 0.1 degree\n<3> C = degrees C\n<4> WCHR (ID indicating relative wind chill)\n<5> C = temperature\n<6> Calculated “theoretical” wind chill temperature, degrees Celsius, to the nearest 0.1 degree\n<7> C = degrees C\n<8> WCHT (ID indicating theoretical wind chill)\n<9> C = temperature\n<10> Calculated heat index, degrees Celsius, to the nearest 0.1 degree (this field left blank by WeatherStation)\n<11> C = degrees C\n<12> HINX (ID indicating heat index)\n<13> P = pressure\n<14> Actual measured barometric pressure, or \"station pressure\", bars, to the nearest 0.001 bar\n<15> B = bars\n<16> STNP (ID indicating station pressure)"
          n140 = call "Airmar Generate RegEx.vi"("# Datums"=16) -> ("RegEx"=w1482:string)
          n141 = xnode "Match Regular Expression"("input string"=w1476, "regular expression"=w1482) -> ("submatch 2"=w1480:string, "submatch 6"=w1479:string, "submatch 10"=w1478:string, "submatch 14"=w1477:string)  [unwired: 4 in, 17 out]
          n142 = Fract/Exp String To Number(string=w1480) -> (number=w1486:dbl)  [unwired: 3 in, 1 out]
          n143 = Fract/Exp String To Number(string=w1479) -> (number=w1485:dbl)  [unwired: 3 in, 1 out]
          n144 = Fract/Exp String To Number(string=w1478) -> (number=w1484:dbl)  [unwired: 3 in, 1 out]
          n145 = Fract/Exp String To Number(string=w1477) -> (number=w1483:dbl)  [unwired: 3 in, 1 out]
          n146 = Bundle By Name(cluster=T12 {"Calc. Relative Wind Chill (degC)"=0.0, "Calc. Theoretical Wind Chill (degC)"=0.0, "Calc. Heat Index (degC)"=0.0, "Meas. Barometric Pressure (bars)"=0.0} ("Transducer (XDR) A Data 2"), "Calc. Relative Wind Chill (degC)"=w1486, "Calc. Theoretical Wind Chill (degC)"=w1485, "Calc. Heat Index (degC)"=w1484, "Meas. Barometric Pressure (bars)"=w1483) -> (→"Transducer (XDR) A Data":T12)
        }
      }
    }
  }
